vi "test-VAttributes-VAttributesToDat(partsOfAttrs).vi"(8 "error in (no error)":errorcluster, 11 "TestCase in":refnum<class "MyTestCase.lvclass">) -> (0 "error out":errorcluster, 3 "TestCase out":refnum<class "MyTestCase.lvclass">)   [LabVIEW 2019, in "MyTestCase.lvclass"]
uses:
  MyTestCase.lvclass
  <vilib>/addons/_JKI Toolkits/VI Tester/TestCase.llb/TestCase.lvclass
  lv-apt-json-file.lvlib
  C:/Program Files (x86)/National Instruments/LabVIEW 2019/vi.lib/addons/_JKI Toolkits/VI Tester/TestCase.llb/TestCase.lvclass
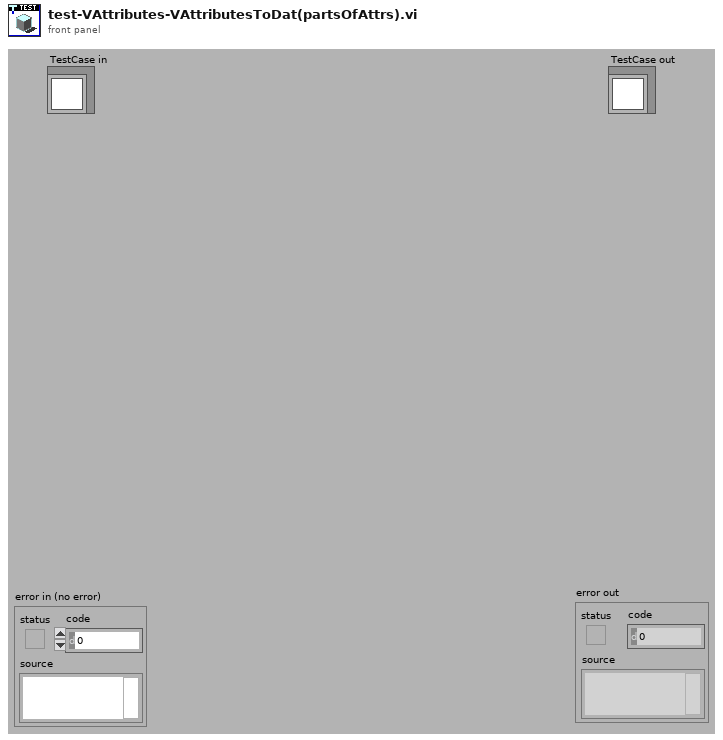
[diagram p1: front panel]
types:
  T1 = cluster{"numeric":i32, "string":string, "Cluster":cluster{"numeric":i32, "string":string, "cluster":cluster{"numeric":i32, "string":string, "cluster":cluster{"numeric":i32, "string":string}}}}
  T2 = cluster{"bool":bool, "string2":string, "cluster":cluster{"cluster2":cluster{"bool":bool}, "numeric":i32, "string":string, "cluster":cluster{"string":string, "numeric":i32}}, "string":string}
  T3 = cluster{"bool":bool, "string2":string, "cluster":cluster{"numeric":i32, "string":string, "cluster":cluster{"numeric":i32, "string":string}}}
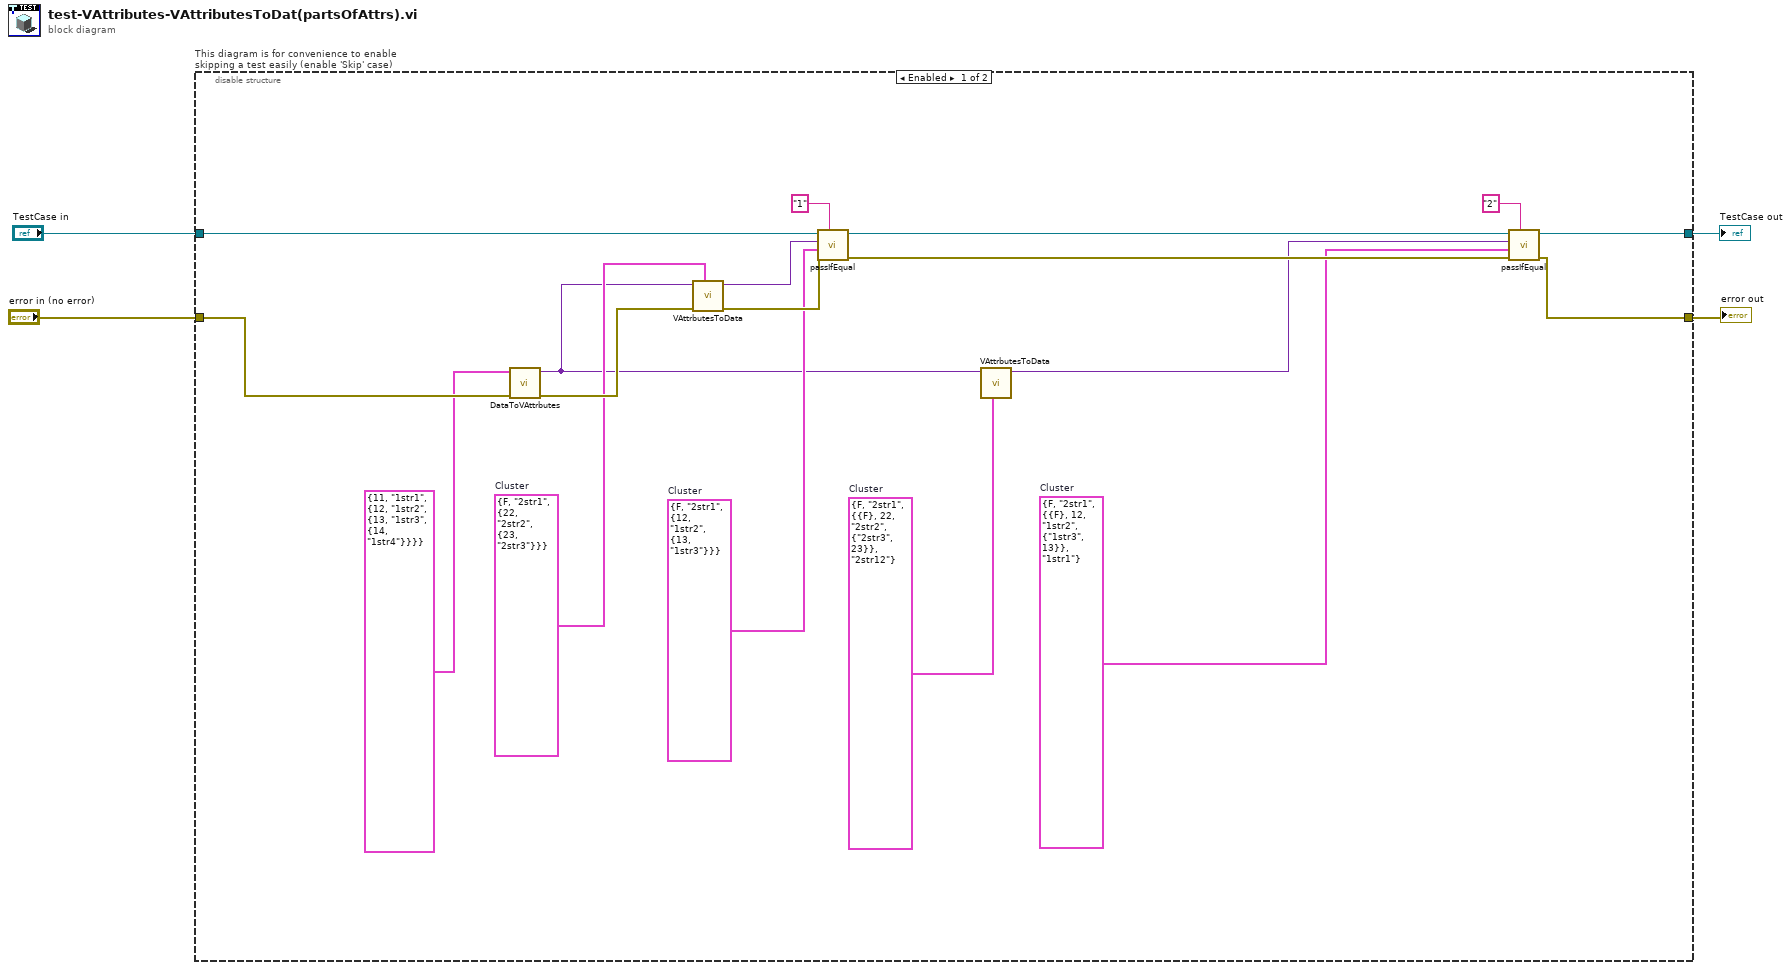
[diagram p0: block diagram]
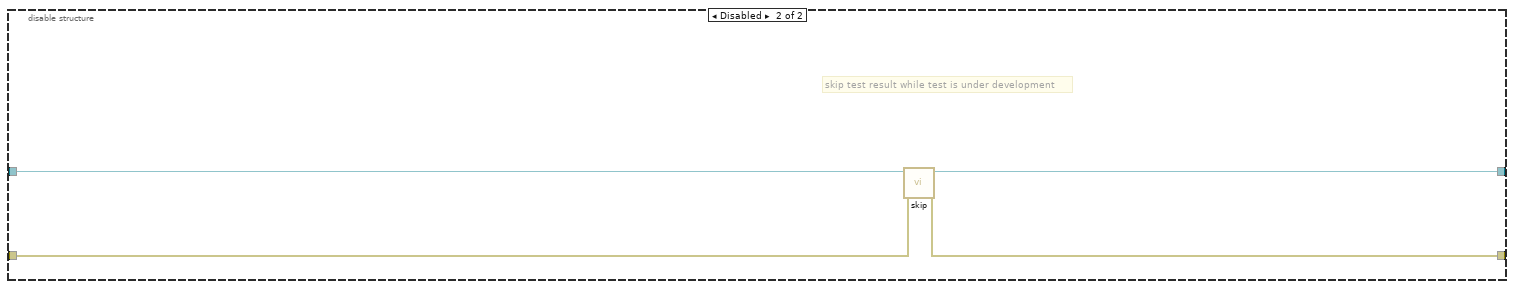
[diagram p2: hidden frame]
diagram:
  n1 = disable-structure "This diagram is for convenience to enable skipping a test easily (enable 'Skip' case)" shown="Enabled" {
    disable-tunnel: "TestCase in" -> [w20 w26]
    disable-tunnel: [w17 w24] -> w1
    disable-tunnel: [w16 w25] -> w3
    disable-tunnel: "error in (no error)" -> [w21 w23]
    frame Enabled {
      w5 = T2 {"bool"=FALSE, "string2"="2str1", "cluster"={"cluster2"={"bool"=FALSE}, "numeric"=12, "string"="1str2", "cluster"={"string"="1str3", "numeric"=13}}, "string"="1str1"}  # Cluster
      w8 = T2 {"bool"=FALSE, "string2"="2str1", "cluster"={"cluster2"={"bool"=FALSE}, "numeric"=22, "string"="2str2", "cluster"={"string"="2str3", "numeric"=23}}, "string"="2str12"}  # Cluster
      w10 = T3 {"bool"=FALSE, "string2"="2str1", "cluster"={"numeric"=12, "string"="1str2", "cluster"={"numeric"=13, "string"="1str3"}}}  # Cluster
      w11 = T3 {"bool"=FALSE, "string2"="2str1", "cluster"={"numeric"=22, "string"="2str2", "cluster"={"numeric"=23, "string"="2str3"}}}  # Cluster
      n2 = call "DataToVAttrbutes.vi"("error in (no error)"=w21, "data"=T1 {"numeric"=11, "string"="1str1", "Cluster"={"numeric"=12, "string"="1str2", "cluster"={"numeric"=13, "string"="1str3", "cluster"={"numeric"=14, "string"="1str4"}}}} ("Cluster")) -> ("error out"=w22:errorcluster, "VAttributes"=w9:variant)  [unwired: 8 in]
      n3 = call "VAttrbutesToData.vi"("Prototype"=w11, "error in (no error)"=w22, "VAttributes"=w9) -> ("error out"=w14:errorcluster, "data"=w12:variant)  [unwired: 7 in]
      n4 = call-dynamic "passIfEqual.vi"("custom report message (\"\")"="1" ("custom report message (\"\")"), "error in (no error)"=w14, "y"=w10, "x"=w12, "TestCase in"=w20) -> ("error out"=w19:errorcluster, "TestCase out"=w18:refnum<class "MyTestCase.lvclass">)  [unwired: 5 in]
      n5 = call "VAttrbutesToData.vi"("Prototype"=w8, "VAttributes"=w9) -> ("data"=w6:variant)  [unwired: 8 in, 1 out]
      n6 = call-dynamic "passIfEqual.vi"("custom report message (\"\")"="2" ("custom report message (\"\")"), "error in (no error)"=w19, "y"=w5, "x"=w6, "TestCase in"=w18) -> ("error out"=w16:errorcluster, "TestCase out"=w17:refnum<class "MyTestCase.lvclass">)  [unwired: 5 in]
    }
    frame Disabled {
      # "skip test result while test is under development"
      n7 = call <vilib>:"skip.vi"("error in (no error)"=w23, "TestCase in"=w26) -> ("error out"=w25:errorcluster, "TestCase out"=w24:refnum<class "MyTestCase.lvclass">)  [unwired: 8 in]
    }
  }
  "error out" <- w3
  "TestCase out" <- w1
